vi "Tab_EventStructure.vi"() -> ()   [LabVIEW 2015]
panel:
  in  "stop":bool
  in  "Tab Control":enum32{"Page 1", "Page 2", "Page 3"}(tab)
  out "Slide":u8(slide) scale=0.0..100.0
  in  "Knob":dbl(knob) scale=0.0..100.0
  out "Tank":dbl(slide) scale=0.0..10.0
  in  "Gauge":dbl(knob) scale=0.0..10.0
  out "Slide 2":u8(slide) scale=0.0..100.0
  in  "Meter":dbl(knob) scale=0.0..100.0
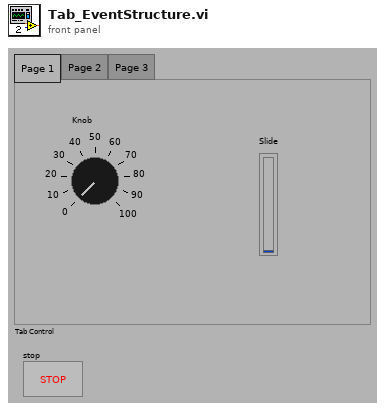
[diagram p1: front panel]
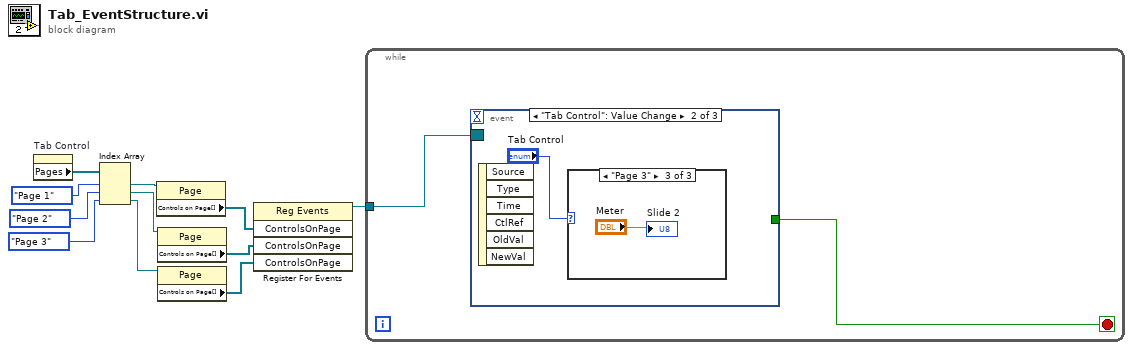
[diagram p0: block diagram]
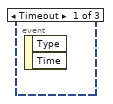
[diagram p2: hidden frame]
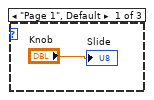
[diagram p3: hidden frame]
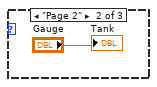
[diagram p4: hidden frame]
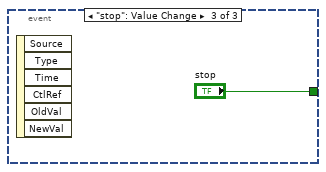
[diagram p5: hidden frame]
diagram:
  n1 = property on="Tab Control" class="TabCtl (strict)"() -> ("Pages"=w11:refnum<vi>[])  [unwired: 2 in, 2 out]
  n2 = Index Array(array=w11, index #1=enum32{"Page 1", "Page 2", "Page 3"}."Page 1" ("Tab Control"), index #2=enum32{"Page 1", "Page 2", "Page 3"}."Page 2" ("Tab Control"), index #3=enum32{"Page 1", "Page 2", "Page 3"}."Page 3" ("Tab Control")) -> (element #1=w7:refnum<vi>, element #2=w6:refnum<vi>, element #3=w5:refnum<vi>)
  n3 = property class="Page"(reference=w7) -> ("Controls on Page[]"=w4:refnum<vi>[])  [unwired: 1 in, 2 out]
  n4 = property class="Page"(reference=w6) -> ("Controls on Page[]"=w3:refnum<vi>[])  [unwired: 1 in, 2 out]
  n5 = property class="Page"(reference=w5) -> ("Controls on Page[]"=w2:refnum<vi>[])  [unwired: 1 in, 2 out]
  n6 = register-events(w4, w3, w2) -> (reference out=w1:refnum<event-registration>)  [unwired: 2 in, 1 out]
  n7 = while {
    tunnel: w1 -> [w12]
    stop <- w13 stop-if-true
    n8 = event shown="[1] \"Tab Control\": Value Change" {
      selector: w12 -> [_ _ _]
      dyn-events: _ -> [_ _ _]
      timeout: _ -> [_ _ _]
      tunnel: [_ _ "stop"] -> w13
      event Timeout {
        n9 = event-data() -> ()  [unwired: 1 in, 2 out]
      }
      event "Tab Control": Value Change {
        n10 = event-data() -> ()  [unwired: 1 in, 6 out]
        n11 = case shown="\"Page 3\"" "Tab Control" {
          frame "Page 1", Default {
            "Slide" <- "Knob"
          }
          frame "Page 2" {
            "Tank" <- "Gauge"
          }
          frame "Page 3" {
            "Slide 2" <- "Meter"
          }
        }
      }
      event "stop": Value Change {
        n12 = event-data() -> ()  [unwired: 1 in, 6 out]
      }
    }
  }
